vi "Send Notification Msg.vi"(8 "error in (no error)":errorcluster, 9 "Publication Time (Use Current Time)":timestamp, 10 "Value":variant, 11 "Notification Msg":refnum<class "Notification Msg.lvclass">) -> (0 "error out":errorcluster)   [LabVIEW 2017, in "Transport.lvlib" / "Notification Msg.lvclass"]
doc: "<License>\nCopyright © 2017 Composed Systems, LLC | All rights reserved\nwww.composed.io\n\nAuthor: Ethan Stern <ethan.stern@composed.io>\n\nThis software is provided \"AS IS\" WITHOUT WARRANTIES, either express or implied, AND IS FOR EDUCATIONAL PURPOSES ONLY.\n</License>"
uses:
  Notification Msg.lvclass
  gpm_packages/@cs/transport/Source/Concrete/ActorMessageTransport/Notification Msg/Notification Msg.lvclass
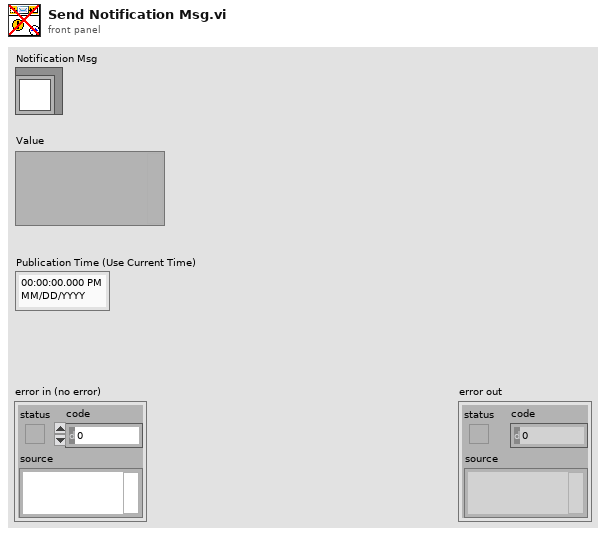
[diagram p1: front panel]
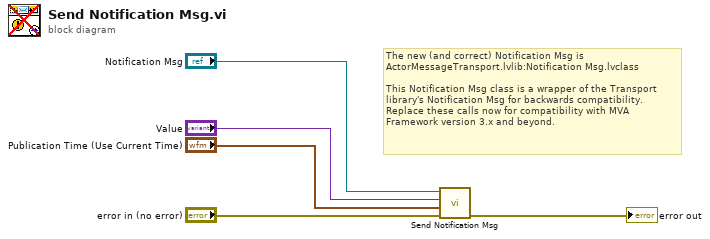
[diagram p0: block diagram]
diagram:
  # "The new (and correct) Notification Msg is\nActorMessageTransport.lvlib:Notification Msg.lvclass\n\nThis Notification Msg class is a wrapper of the Transport\nlibrary's Notification Msg for backwards compatibility.\nReplace these calls now for compatibility with MVA\nFramework version 3.x and beyond."
  n1 = call-parent "Send Notification Msg.vi"("error in (no error)"="error in (no error)", "Publication Time (Use Current Time)"="Publication Time (Use Current Time)", "Value"="Value", "Notification Msg"="Notification Msg") -> ("error out"=→"error out":errorcluster)  [unwired: 7 in]
